vi "Build Relation Query String.vi"(5 "Related To Table Name":string, 7 "Reversed By Column Name":string, 8 "error in (no error)":errorcluster, 9 "Types":refnum<class "Type.lvclass">[](array[class]), 10 "From Mapping":T1, 11 "SQLite in":refnum<class "SQLite.lvclass">) -> (0 "error out":errorcluster, 2 "Query String":string)   [LabVIEW 2020, in "Conditum SQLite.lvlib" / "SQLite.lvclass"]
uses:
  SQLite.lvclass
  <vilib>/IlluminatedG/IG Conditum Base/Conditum/Relation Mapping.ctl
  <vilib>/IlluminatedG/IG Conditum Base/Conditum/Columns/Type/Type.lvclass
  <vilib>/IlluminatedG/IG Conditum Base/Conditum/Columns/Type/Type.lvclass/Type.ctl
  SQLite.lvclass/SQLite.ctl
  <vilib>/IlluminatedG/IG Conditum Base/Conditum/Conditum.lvlib
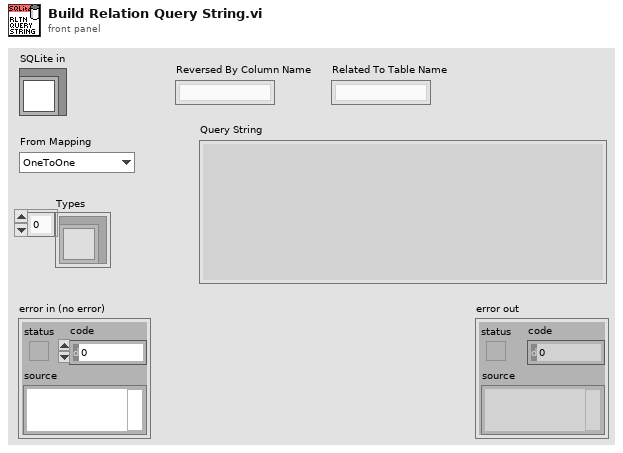
[diagram p1: front panel]
types:
  T1 = typedef "Conditum.lvlib/Relation Mapping.ctl" = enum16{"OneToOne", "OneToMany", "ManyToOne", "ManyToMany"}
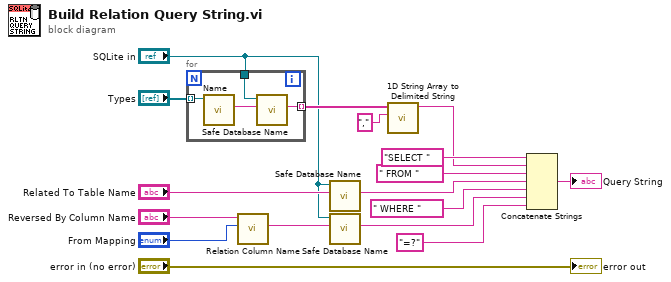
[diagram p0: block diagram]
diagram:
  n1 = for {
    tunnel: "Types" -> [w21] mode=indexing
    tunnel: [w19] -> w16 mode=indexing
    tunnel: "SQLite in" -> [w18]
    n2 = call <vilib>:"Name.vi"("Type in"=w21) -> ("Table Name"=w20:string)  [unwired: 10 in]
    n3 = call-dynamic "Safe Database Name.vi"("Conditum Name"=w20, "Database in"=w18) -> ("Database Name"=w19:string)  [unwired: 9 in]
  }
  n4 = call "Relation Column Name.vi"("From Mapping"="From Mapping", "Reverse by Name"="Reversed By Column Name") -> ("Column Name"=w6:string)  [unwired: 9 in]
  n5 = call-dynamic "Safe Database Name.vi"("Conditum Name"="Related To Table Name", "Database in"="SQLite in") -> ("Database Name"=w3:string)  [unwired: 9 in]
  n6 = call-dynamic "Safe Database Name.vi"("Conditum Name"=w6, "Database in"="SQLite in") -> ("Database Name"=w2:string)  [unwired: 9 in]
  n7 = call <vilib>:"1D String Array to Delimited String.vi"("delimiter"=",", "string array"=w16) -> ("delimited string"=w12:string)  [unwired: 9 in]
  n8 = Concatenate Strings("SELECT ", w12, " FROM ", w3, " WHERE ", w2, "=?") -> (→"Query String":string)
  "error out" <- "error in (no error)"
